vi "DynamicUI.vi"(8 "error in (no error)":errorcluster, 11 "Numeric in":refnum<class "Numeric.lvclass">) -> (0 "error out":errorcluster, 3 "Numeric out":refnum<class "Numeric.lvclass">)   [LabVIEW 2023, in "Numeric.lvclass"]
uses:
  Numeric.lvclass
panel:
  out "Numeric Data":dbl
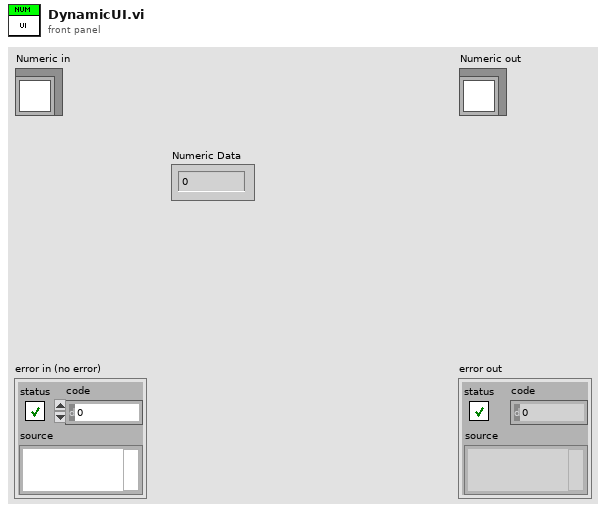
[diagram p1: front panel]
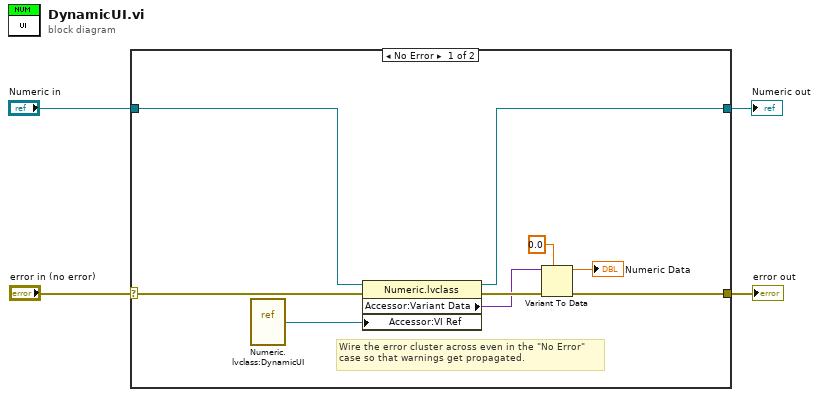
[diagram p0: block diagram]
diagram:
  n1 = case shown="No Error" "error in (no error)" {
    selector: "error in (no error)" -> [w13 w15]
    tunnel: [w9 w15] -> w3
    tunnel: [w10 w14] -> w1
    tunnel: "Numeric in" -> [w11 w14]
    frame No Error {
      # "Wire the error cluster across even in the \"No Error\"\ncase so that warnings get propagated."
      n2 = vi-ref "Numeric.lvclass:DynamicUI.vi"() -> (w5:refnum<vi>)
      n3 = property class="Numeric.lvclass"(reference=w11, error in=w13, "Accessor:VI Ref"=w5) -> (reference out=w10:refnum<class "Numeric.lvclass">, error out=w12:errorcluster, "Accessor:Variant Data"=w8:variant)
      n4 = Variant To Data(error in=w12, type=0.0, Variant=w8) -> (data=→"Numeric Data":dbl, error out=w9:errorcluster)
    }
    frame Error {
    }
  }
  "error out" <- w3
  "Numeric out" <- w1
